vi "in_interior slope.vi"(10 "h[0..1]":dbl[](array[numeric]) format="%_6g", 11 "delta[0..1]":dbl[](array[numeric]) format="%_6g") -> (3 "interior slope":dbl format="%_6g")   [LabVIEW 2011, in "NI_Gmath.lvlib"]
uses:
  NI_Gmath.lvlib
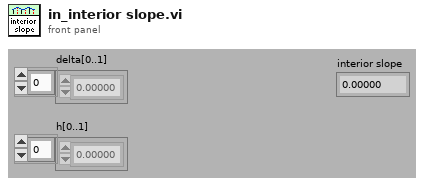
[diagram p1: front panel]
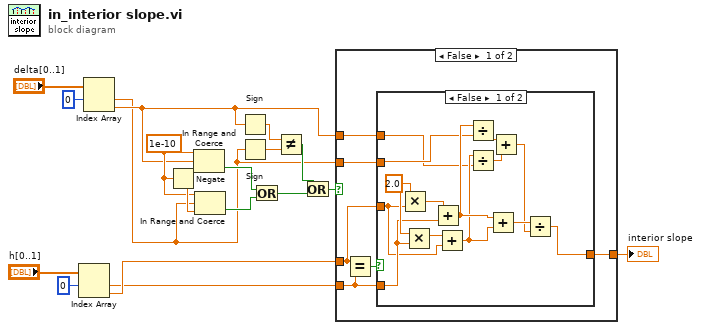
[diagram p0: block diagram]
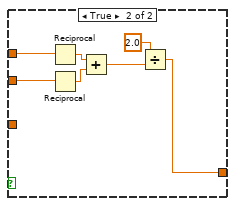
[diagram p2: hidden frame]
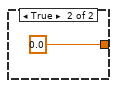
[diagram p3: hidden frame]
diagram:
  w9 = 1e-10 ("upper limit")
  n1 = Index Array(array="h[0..1]", index #1=0 ("index")) -> (element #1=w4:dbl, element #2=w5:dbl)  [unwired: 1 in]
  n2 = Index Array(array="delta[0..1]", index #1=0 ("index")) -> (element #1=w1:dbl, element #2=w3:dbl)  [unwired: 1 in]
  n3 = Negate(x=w9) -> (-x=w10:dbl)
  n4 = In Range and Coerce(upper limit=w9, x=w3, lower limit=w10) -> (In Range?=w7:bool)  [unwired: 1 out]
  n5 = In Range and Coerce(upper limit=w9, x=w1, lower limit=w10) -> (In Range?=w8:bool)  [unwired: 1 out]
  n6 = Sign(1:w3) -> (0:w14:dbl)
  n7 = Sign(1:w1) -> (0:w13:dbl)
  n8 = Or(x=w7, y=w8) -> (x .or. y?=w6:bool)
  n9 = Not Equal?(x=w14, y=w13) -> (x != y?=w12:bool)
  n10 = Or(x=w12, y=w6) -> (x .or. y?=w11:bool)
  n11 = case shown="False" w11 {
    tunnel: [w21 0.0] -> w2
    tunnel: w5 -> [w20 _]
    tunnel: w4 -> [w19 _]
    tunnel: w1 -> [w22 _]
    tunnel: w3 -> [w23 _]
    frame False {
      n12 = Equal?(x=w20, y=w19) -> (x = y?=w24:bool)
      n13 = case shown="False" w24 {
        tunnel: w23 -> [w26 w45]
        tunnel: w22 -> [w27 w44]
        tunnel: [w28 w39] -> w21
        tunnel: w20 -> [w34 _]
        tunnel: w19 -> [w35 _]
        frame False {
          w36 = 2.0 ("x")
          n14 = Multiply(x=w36, y=w34) -> (x*y=w25:dbl)
          n15 = Multiply(x=w36, y=w35) -> (x*y=w33:dbl)
          n16 = Add(x=w25, y=w35) -> (x+y=w32:dbl)
          n17 = Add(x=w33, y=w34) -> (x+y=w31:dbl)
          n18 = Divide(x=w32, y=w27) -> (x/y=w37:dbl)
          n19 = Divide(x=w31, y=w26) -> (x/y=w38:dbl)
          n20 = Add(x=w32, y=w31) -> (x+y=w30:dbl)
          n21 = Add(x=w37, y=w38) -> (x+y=w29:dbl)
          n22 = Divide(x=w30, y=w29) -> (x/y=w28:dbl)
        }
        frame True {
          n23 = Reciprocal(x=w45) -> (1/x=w43:dbl)
          n24 = Reciprocal(x=w44) -> (1/x=w42:dbl)
          n25 = Add(x=w43, y=w42) -> (x+y=w40:dbl)
          n26 = Divide(x=2.0, y=w40) -> (x/y=w39:dbl)
        }
      }
    }
    frame True {
    }
  }
  "interior slope" <- w2
